vi "SprawdzPozycje.vi"(8 "error in (no error)":errorcluster, 9 "Car Position Slider":u8, 10 "Job Array Index":i32, 11 "Job Array":T1[](array[typedef])) -> (0 "error out":errorcluster, 3 "Car Out of Position?":bool)   [LabVIEW 2012]
doc: "Author: Alex Anderson\nDate: 2/6/2013\n\nThis VI Indexes out the current job and checks it's required\nposition against the state of the car position slider. Don't bother\nif error present as I intend the code to shut down in the presence\nof an error.\n\nThe position slider should really be an enum as well. As it stands\nI'm relying on no one reordering the Positions on the slider."
uses:
  Controls/Wash Step Info.ctl
  Controls/Wash Step Enum.ctl
  Controls/Station Enum.ctl
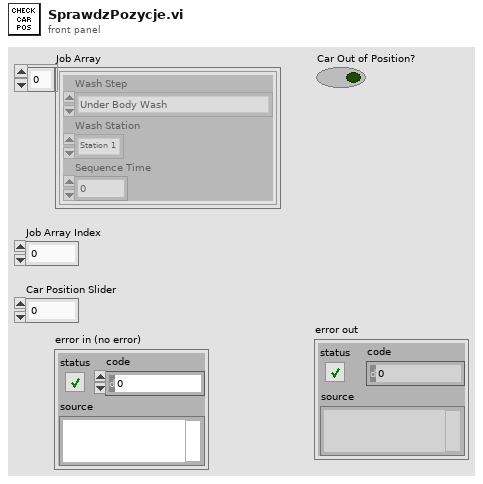
[diagram p1: front panel]
types:
  T1 = typedef "Wash Step Info.ctl" = cluster{"Wash Step":T2, "Wash Station":T3, "Sequence Time":dbl}
  T2 = typedef "Wash Step Enum.ctl" = enum16{"Under Body Wash", "Bug Remover", "Pre-Soak", "High Pressure Wash", "Low Pressure Wax", "Spot Free Rinse", "Tire Shine Foam", "Air Dry", "Exiting"}
  T3 = typedef "Station Enum.ctl" = enum16{"Entry", "Station 1", "Station 2", "Station 3", "Exit"}
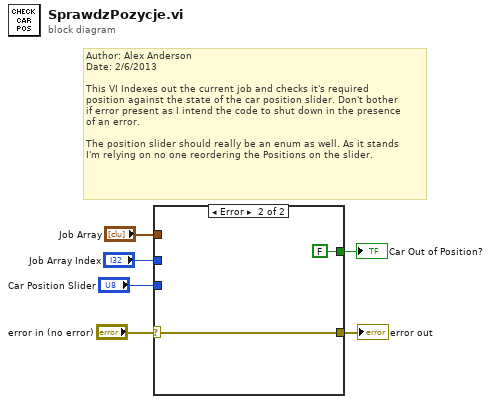
[diagram p0: block diagram]
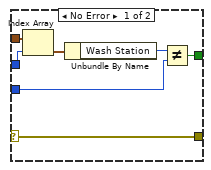
[diagram p2: hidden frame]
diagram:
  # "Author: Alex Anderson\nDate: 2/6/2013\n\nThis VI Indexes out the current job and checks it's required\nposition against the state of the car position slider. Don't bother\nif error present as I intend the code to shut down in the presence\nof an error.\n\nThe position slider should really be an enum as well. As it stands\nI'm relying on no one reordering the Positions on the slider."
  n1 = case shown="Error" "error in (no error)" {
    selector: "error in (no error)" -> [w7 w14]
    tunnel: "Job Array Index" -> [w13 _]
    tunnel: [w12 FALSE] -> w5
    tunnel: "Job Array" -> [w9 _]
    tunnel: "Car Position Slider" -> [w8 _]
    tunnel: [w7 w14] -> w1
    frame No Error {
      n2 = Index Array(array=w9, index=w13) -> (element=w10:T1)
      n3 = Unbundle By Name(w10) -> ("Wash Station"=w11:T3)
      n4 = Not Equal?(x=w11, y=w8) -> (x != y?=w12:bool)
    }
    frame Error {
    }
  }
  "Car Out of Position?" <- w5
  "error out" <- w1
